vi "Check Can Destroy.vi"(8 "Error in":errorcluster, 10 "Actor in":refnum<class "Actor.lvclass">) -> (1 "Destroy":bool, 2 "Actor out":refnum<class "Actor.lvclass">)   [LabVIEW 2020, in "jettl.lvlib" / "Actor.lvlib"]
uses:
  Actor.lvlib
  Actor/Actor.lvclass
  Go To Destroy Msg/Go To Destroy Msg.lvlib
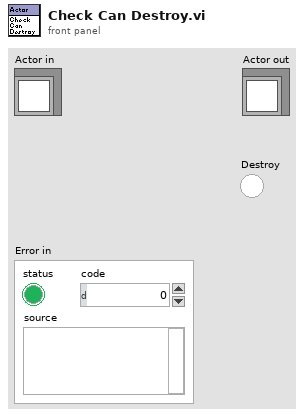
[diagram p1: front panel]
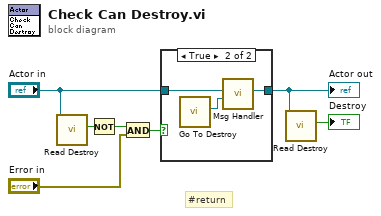
[diagram p0: block diagram]
diagram:
  # "#return"
  n1 = call-dynamic "Read Destroy.vi"("Actor in"="Actor in") -> ("Destroy"=w5:bool)  [unwired: 10 in]
  n2 = Not(x=w5) -> (.not. x?=w4:bool)
  n3 = And(x=w4, y="Error in") -> (x .and. y?=w3:bool)
  n4 = case shown="True" w3 {
    tunnel: "Actor in" -> [w8 w11]
    tunnel: [w8 w9] -> w2
    frame False {
    }
    frame True {
      n5 = call "Go To Destroy.vi"() -> ("Msg"=w10:refnum<class "Msg.lvclass">)  [unwired: 11 in]
      n6 = call "Msg Handler.vi"("Msg"=w10, "Actor in"=w11) -> ("Actor out"=w9:refnum<class "Actor.lvclass">)  [unwired: 8 in, 1 out]
    }
  }
  "Actor out" <- w2
  n7 = call-dynamic "Read Destroy.vi"("Actor in"=w2) -> ("Destroy"=→"Destroy":bool)  [unwired: 10 in]
